vi "Controller Module.vi"(8 "error in":errorcluster) -> (0 "error out":errorcluster)   [LabVIEW 2025, in "Contoller.lvlib"]
doc: "This is the top level module for the ATM controller. \n\nIt is closed using a user event. It communicates with the other modules using aqueue based API which has comms modules that can be swapped if required."
uses:
  Contoller.lvlib
  Private Controls/Module Data Cluster.ctl
  Error Handler/Error Handler.lvlib
  Display/Display Console/Display Console.lvlib
  Public Control/ATM Transactions.ctl
  Private Controls/Control_Data.ctl
  Sensor/Sensor Console/Sensor Console.lvlib
  Simulated Console (UI)/Simulated Console.lvlib
  Config DataBase/Config Database.lvlib
  User Events/Controls/UE Abort Action.ctl
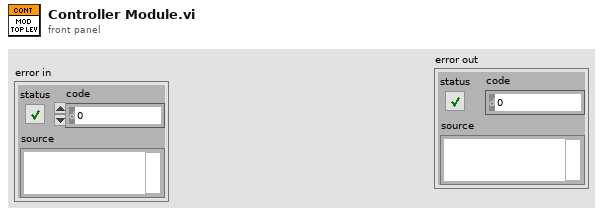
[diagram p1: front panel]
types:
  T1 = typedef "Contoller.lvlib/Control_Data.ctl" = cluster{"Transactions":T2, "Number Log Ins":dbl}
  T2 = typedef "Contoller.lvlib/ATM Transactions.ctl" = enum16{"Welcome", "Login", "Idle ", "Invalid Login", "Terminate Session", "Deposit", "Withdrawal", "Fast Cash", "Withdrawal Complete", "Withdrawal Failed", "Balance Inquiry"}
  T3 = typedef "Contoller.lvlib/Module Data Cluster.ctl" = cluster{"Data":variant, "Action":enum16{"Log In Init", "Fast Cash", "New transaction", "Withdrawal Init", "Recieve Keypad", "Deposit Finish", "Balance", "Withdrawal Approved", "Terminate", "Deposit Init", "Error", "Exit", "Init", "Log In Finish", "Cancel Transaction", "Withdrawal Failed", "Cash Removed"}}
  T4 = typedef "UE Abort Action.ctl" = enum16{"Destroy", "Get", "Create"}
  T5 = enum16{"Log In Init", "Fast Cash", "New transaction", "Withdrawal Init", "Recieve Keypad", "Deposit Finish", "Balance", "Withdrawal Approved", "Terminate", "Deposit Init", "Error", "Exit", "Init", "Log In Finish", "Cancel Transaction", "Withdrawal Failed", "Cash Removed"}
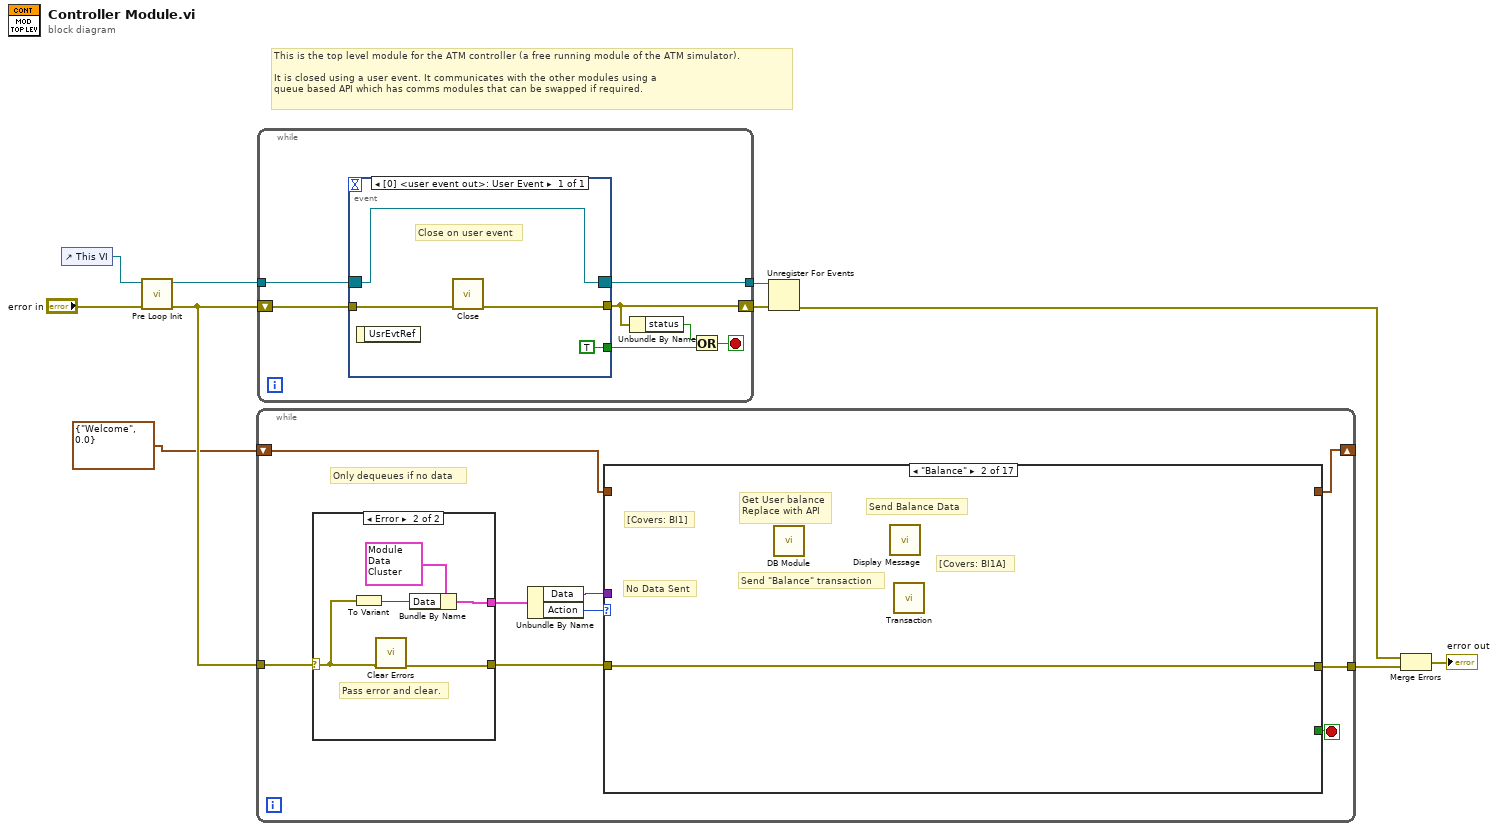
[diagram p0: block diagram]
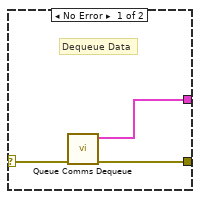
[diagram p2: hidden frame]
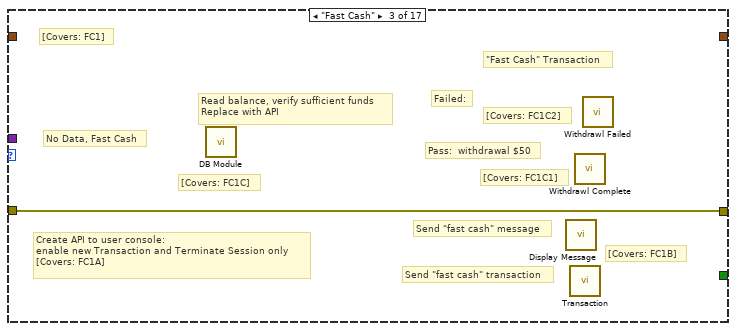
[diagram p4: hidden frame]
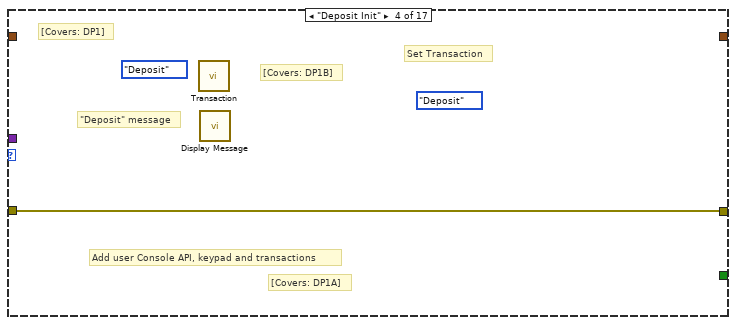
[diagram p5: hidden frame]
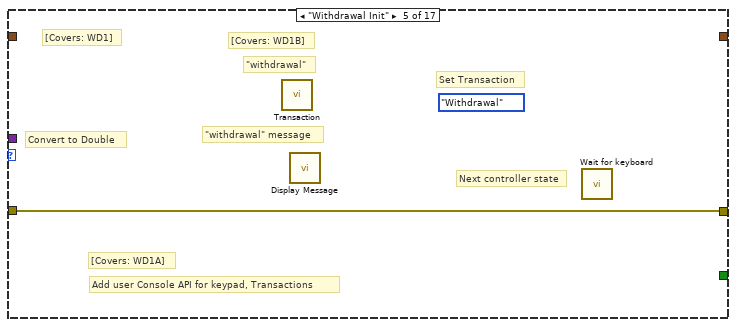
[diagram p6: hidden frame]
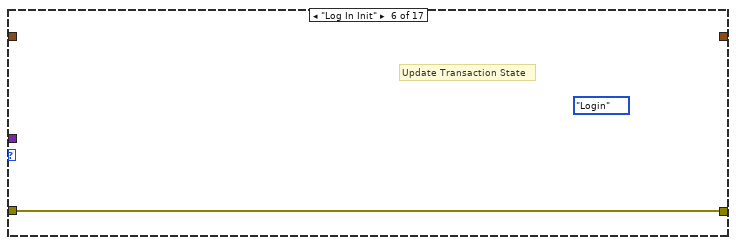
[diagram p7: hidden frame]
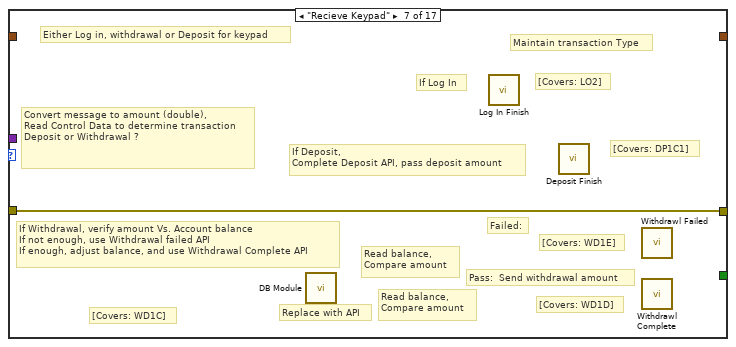
[diagram p8: hidden frame]
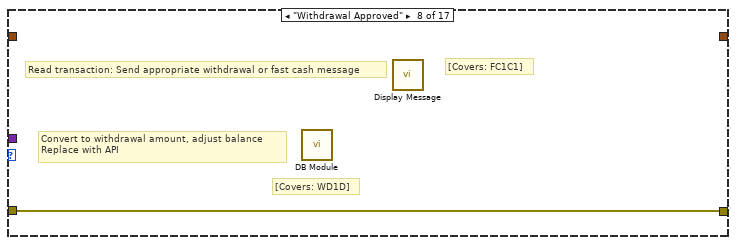
[diagram p9: hidden frame]
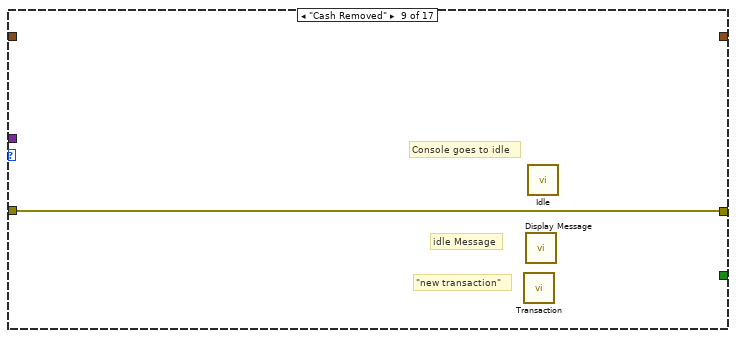
[diagram p10: hidden frame]
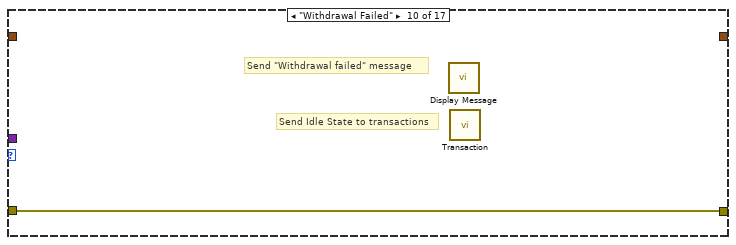
[diagram p11: hidden frame]
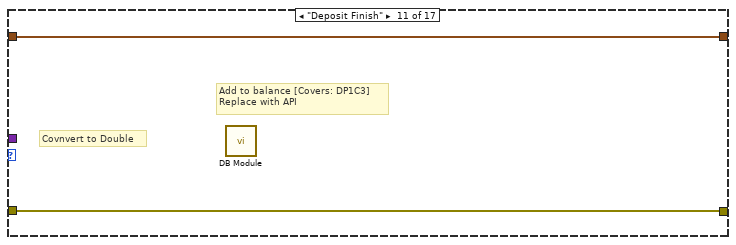
[diagram p12: hidden frame]
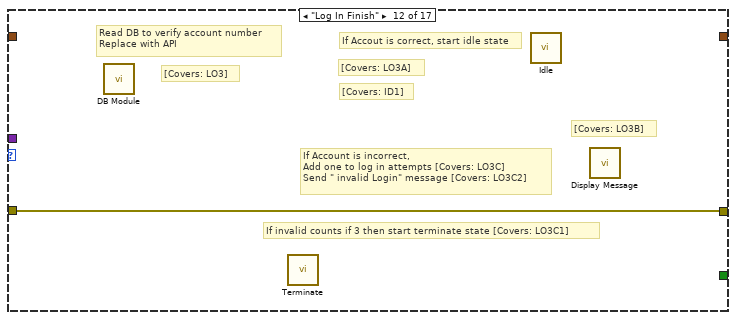
[diagram p13: hidden frame]
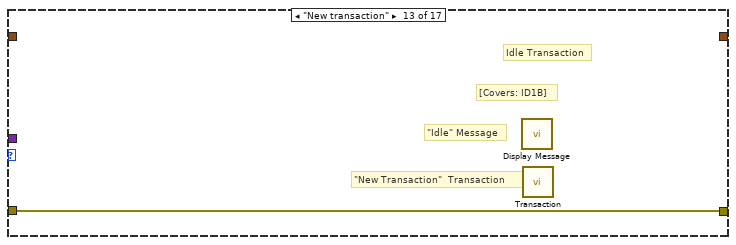
[diagram p14: hidden frame]
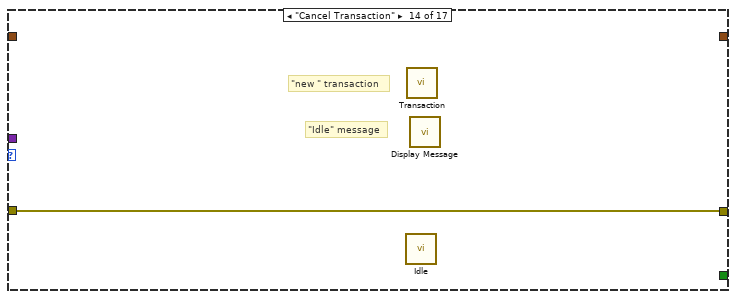
[diagram p15: hidden frame]
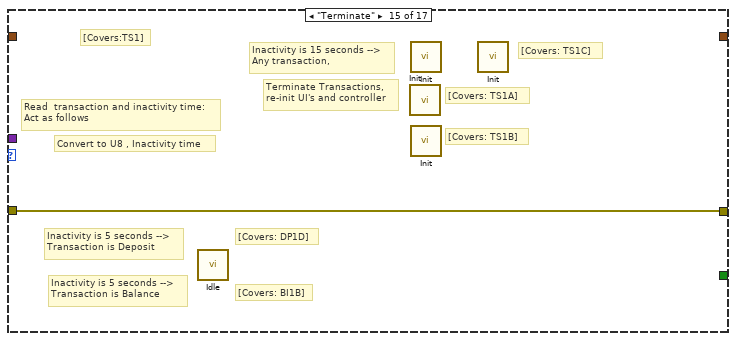
[diagram p16: hidden frame]
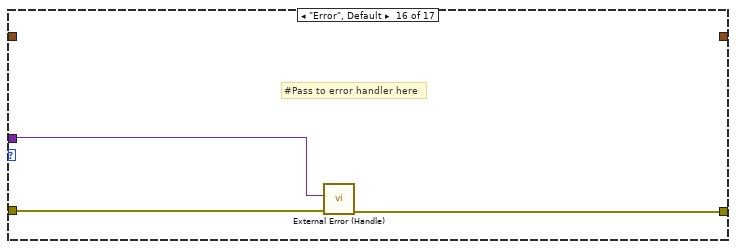
[diagram p17: hidden frame]
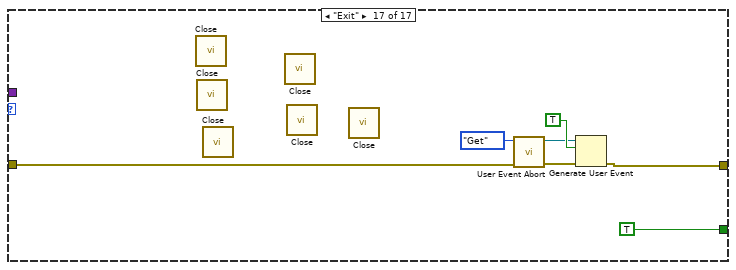
[diagram p18: hidden frame]
diagram:
  # "This is the top level module for the ATM controller (a free running module of the ATM simulator). \n\nIt is closed using a user event. It communicates with the other modules using a\nqueue based API which has comms modules that can be swapped if required."
  n1 = control-ref of="This VI"() -> (w10:refnum<vi>)
  n2 = call "Pre Loop Init.vi"("error in"="error in", "Ref In"=w10) -> ("error out"=w5:errorcluster, "Event Registration Refnum"=w8:refnum<event-registration>)  [unwired: 8 in]
  n3 = while {
    tunnel: w5 -> [w18]
    tunnel: [w13] -> w3
    shift-right: [w11] -> _
    shift-left: T1 {"Transactions"=enum."Welcome", "Number Log Ins"=0.0} ("Control_Data") -> [w12]
    stop <- w19 stop-if-true
    # "Only dequeues if no data"
    n4 = case shown="Error" w18 {
      selector: w18 -> [w21 w24]
      tunnel: [w22 w23] -> w16
      tunnel: [w20 w25] -> w17
      frame No Error {
        # "Dequeue Data"
        n5 = call "Queue Comms Dequeue.vi"("error in"=w21) -> ("error out"=w22:errorcluster, "Data Out"=w20:T3)  [unwired: 9 in]
      }
      frame Error {
        # "Pass error and clear."
        n6 = To Variant(anything=w24) -> (Variant=w26:variant)
        n7 = call <vilib>:"Clear Errors.vi"("error in (no error)"=w24) -> ("error out"=w23:errorcluster)  [unwired: 5 in, 1 out]
        n8 = Bundle By Name(cluster=T3 {"Data"=variant, "Action"=enum."Error"} ("Cluster"), "Data"=w26) -> (w25:T3)
      }
    }
    n9 = Unbundle By Name(w17) -> ("Data"=w14:variant, "Action"=w15:T5)
    n10 = case shown="\"Balance\"" w15 {
      tunnel: [_ _ _ _ _ _ _ _ _ _ _ _ _ _ _ _ TRUE] -> w19
      tunnel: w16 -> [w28 w29 w30 w31 w32 w33 w34 w35 w36 w37 w39 w40 w41 w42 w43 w45 w48]
      tunnel: w14 -> [_ _ _ _ _ _ _ _ _ _ _ _ _ _ _ w46 _]
      tunnel: [w28 w29 w30 w31 w32 w33 w34 w35 w36 w37 w39 w40 w41 w42 w43 w44 w47] -> w13
      tunnel: w12 -> [_ _ _ _ _ _ _ _ _ _ w38 _ _ _ _ _ _]
      tunnel: [_ _ _ _ _ _ _ _ _ _ w38 _ _ _ _ _ _] -> w11
      frame "Init" {
        # "Set Transaction to Init\nSet Log in attempts to 0"
      }
      frame "Balance" {
        # "[Covers: BI1A]"
        # "Send Balance Data"
        # "Send \"Balance\" transaction"
        # "Get User balance\nReplace with API"
        # "No Data Sent"
        # "[Covers: BI1]"
        n11 = call "DB Module.vi"() -> ()  [unwired: 11 in, 1 out]
        n12 = call "Display Message.vi"() -> ()  [unwired: 11 in, 1 out]
        n13 = call "Transaction.vi"() -> ()  [unwired: 11 in, 1 out]
      }
      frame "Fast Cash" {
        # "[Covers: FC1]"
        # "[Covers: FC1B]"
        # "Send \"fast cash\" transaction"
        # "Send \"fast cash\" message"
        # "\"Fast Cash\" Transaction"
        # "Create API to user console: \nenable new Transaction and Terminate Session only\n[Covers: FC1A]"
        # "[Covers: FC1C]"
        # "Failed:"
        # "[Covers: FC1C2]"
        # "[Covers: FC1C1]"
        # "Pass:  withdrawal $50"
        # "Read balance, verify sufficient funds\nReplace with API"
        # "No Data, Fast Cash"
        n14 = call "DB Module.vi"() -> ()  [unwired: 11 in, 1 out]
        n15 = call "Display Message.vi"() -> ()  [unwired: 11 in, 1 out]
        n16 = call "Transaction.vi"() -> ()  [unwired: 11 in, 1 out]
        n17 = call "Withdrawl Complete.vi"() -> ()  [unwired: 11 in, 1 out]
        n18 = call "Withdrawl Failed.vi"() -> ()  [unwired: 11 in, 1 out]
      }
      frame "Deposit Init" {
        (unwired) ATM_Transactions."Deposit" ("Transactions")
        (unwired) ATM_Transactions."Deposit" ("Transactions")
        # "[Covers: DP1]"
        # "Set Transaction"
        # "Add user Console API, keypad and transactions"
        # "[Covers: DP1A]"
        # "[Covers: DP1B]"
        # "\"Deposit\" message"
        n19 = call "Transaction.vi"() -> ()  [unwired: 11 in, 1 out]
        n20 = call "Display Message.vi"() -> ()  [unwired: 11 in, 1 out]
      }
      frame "Withdrawal Init" {
        (unwired) ATM_Transactions."Withdrawal" ("Transactions")
        # "[Covers: WD1]"
        # "Convert to Double"
        # "Next controller state"
        # "Add user Console API for keypad, Transactions"
        # "[Covers: WD1A]"
        # "Set Transaction"
        # "[Covers: WD1B]"
        # "\"withdrawal\""
        # "\"withdrawal\" message"
        n21 = call "Transaction.vi"() -> ()  [unwired: 11 in, 1 out]
        n22 = call "Display Message.vi"() -> ()  [unwired: 11 in, 1 out]
        n23 = call "Wait for keyboard.vi"() -> ()  [unwired: 11 in, 1 out]
      }
      frame "Log In Init" {
        (unwired) ATM_Transactions."Login" ("Transactions")
        # "Update Transaction State"
      }
      frame "Recieve Keypad" {
        # "Replace with API"
        # "Read balance,\nCompare amount"
        # "[Covers: WD1C]"
        # "[Covers: LO2]"
        # "If Log In"
        # "Failed:"
        # "[Covers: DP1C1]"
        # "Either Log in, withdrawal or Deposit for keypad"
        # "Maintain transaction Type"
        # "[Covers: WD1E]"
        # "[Covers: WD1D]"
        # "Read balance,\nCompare amount"
        # "Pass:  Send withdrawal amount"
        # "If Deposit, \nComplete Deposit API, pass deposit amount"
        # "If Withdrawal, verify amount Vs. Account balance\nIf not enough, use Withdrawal failed API\nIf enough, adjust balance, and use Withdrawal Complete API"
        # "Convert message to amount (double),\nRead Control Data to determine transaction\nDeposit or Withdrawal ?"
        n24 = call "DB Module.vi"() -> ()  [unwired: 11 in, 1 out]
        n25 = call "Log In Finish.vi"() -> ()  [unwired: 11 in, 1 out]
        n26 = call "Deposit Finish.vi"() -> ()  [unwired: 11 in, 1 out]
        n27 = call "Withdrawl Failed.vi"() -> ()  [unwired: 11 in, 1 out]
        n28 = call "Withdrawl Complete.vi"() -> ()  [unwired: 11 in, 1 out]
      }
      frame "Withdrawal Approved" {
        # "[Covers: FC1C1]"
        # "Read transaction: Send appropriate withdrawal or fast cash message"
        # "[Covers: WD1D]"
        # "Convert to withdrawal amount, adjust balance\nReplace with API"
        n29 = call "DB Module.vi"() -> ()  [unwired: 11 in, 1 out]
        n30 = call "Display Message.vi"() -> ()  [unwired: 11 in, 1 out]
      }
      frame "Cash Removed" {
        # "Console goes to idle"
        # "idle Message"
        # "\"new transaction\""
        n31 = call "Transaction.vi"() -> ()  [unwired: 11 in, 1 out]
        n32 = call "Display Message.vi"() -> ()  [unwired: 11 in, 1 out]
        n33 = call "Idle.vi"() -> ()  [unwired: 11 in, 1 out]
      }
      frame "Withdrawal Failed" {
        # "Send Idle State to transactions"
        # "Send \"Withdrawal failed\" message"
        n34 = call "Display Message.vi"() -> ()  [unwired: 11 in, 1 out]
        n35 = call "Transaction.vi"() -> ()  [unwired: 11 in, 1 out]
      }
      frame "Deposit Finish" {
        # "Add to balance [Covers: DP1C3]\nReplace with API"
        # "Covnvert to Double"
        n36 = call "DB Module.vi"() -> ()  [unwired: 11 in, 1 out]
      }
      frame "Log In Finish" {
        # "[Covers: ID1]"
        # "If invalid counts if 3 then start terminate state [Covers: LO3C1]"
        # "[Covers: LO3B]"
        # "If Account is incorrect, \nAdd one to log in attempts [Covers: LO3C] \nSend \" invalid Login\" message [Covers: LO3C2]"
        # "[Covers: LO3A]"
        # "If Accout is correct, start idle state"
        # "[Covers: LO3]"
        # "Read DB to verify account number\nReplace with API"
        n37 = call "DB Module.vi"() -> ()  [unwired: 11 in, 1 out]
        n38 = call "Terminate.vi"() -> ()  [unwired: 11 in, 1 out]
        n39 = call "Idle.vi"() -> ()  [unwired: 11 in, 1 out]
        n40 = call "Display Message.vi"() -> ()  [unwired: 11 in, 1 out]
      }
      frame "New transaction" {
        # "Idle Transaction"
        # "\"Idle\" Message"
        # "\"New Transaction\"  Transaction"
        # "[Covers: ID1B]"
        n41 = call "Display Message.vi"() -> ()  [unwired: 11 in, 1 out]
        n42 = call "Transaction.vi"() -> ()  [unwired: 11 in, 1 out]
      }
      frame "Cancel Transaction" {
        # "\"Idle\" message"
        # "\"new \" transaction"
        n43 = call "Idle.vi"() -> ()  [unwired: 11 in, 1 out]
        n44 = call "Transaction.vi"() -> ()  [unwired: 11 in, 1 out]
        n45 = call "Display Message.vi"() -> ()  [unwired: 11 in, 1 out]
      }
      frame "Terminate" {
        # "[Covers:TS1]"
        # "Inactivity is 5 seconds -->\nTransaction is Balance"
        # "[Covers: BI1B]"
        # "[Covers: DP1D]"
        # "Inactivity is 5 seconds -->\nTransaction is Deposit"
        # "Inactivity is 15 seconds -->\nAny transaction,"
        # "Convert to U8 , Inactivity time"
        # "Read  transaction and inactivity time:\nAct as follows"
        # "[Covers: TS1C]"
        # "[Covers: TS1B]"
        # "[Covers: TS1A]"
        # "Terminate Transactions, \nre-init UI's and controller"
        n46 = call "Idle.vi"() -> ()  [unwired: 11 in, 1 out]
        n47 = call "Init.vi"() -> ()  [unwired: 11 in, 1 out]
        n48 = call "Init.vi"() -> ()  [unwired: 11 in, 1 out]
        n49 = call "Init.vi"() -> ()  [unwired: 11 in, 1 out]
        n50 = call "Init.vi"() -> ()  [unwired: 11 in, 1 out]
      }
      frame "Error", Default {
        # "#Pass to error handler here"
        n51 = call "External Error (Handle).vi"("error in"=w45, "Data"=w46) -> ("error out"=w44:errorcluster)  [unwired: 9 in]
      }
      frame "Exit" {
        n52 = call "Close.vi"() -> ()  [unwired: 11 in, 1 out]
        n53 = call "Close.vi"() -> ()  [unwired: 11 in, 1 out]
        n54 = call "Close.vi"() -> ()  [unwired: 11 in, 1 out]
        n55 = call "Close.vi"() -> ()  [unwired: 11 in, 1 out]
        n56 = call "Close.vi"() -> ()  [unwired: 11 in, 1 out]
        n57 = call "Close.vi"() -> ()  [unwired: 11 in, 1 out]
        n58 = call "User Event Abort.vi"("error in"=w48, "Action"=UE_Abort_Action."Get") -> ("error out"=w50:errorcluster, "user event out"=w51:refnum<user-event>)  [unwired: 8 in]
        n59 = Generate User Event(user event=w51, event data cluster=TRUE ("event data"), error in=w50) -> (error out=w47:errorcluster)  [unwired: 1 in, 1 out]
      }
    }
  }
  n60 = while {
    shift-right: [w57] -> w7
    shift-left: w5 -> [w60]
    tunnel: w8 -> [w55]
    tunnel: [w54] -> w6
    stop <- w58 stop-if-true
    n61 = event shown="[0] <user event out>: User Event" {
      selector: w55 -> [w64]
      dyn-events: [w64] -> w54
      timeout: _ -> [_]
      tunnel: w60 -> [w63]
      tunnel: [w62] -> w57
      tunnel: [TRUE ("stop")] -> w59
      event User Event {
        # "Close on user event"
        n62 = event-data() -> ()  [unwired: 1 in, 1 out]
        n63 = call "Close.vi"("error in"=w63) -> ("error out"=w62:errorcluster)  [unwired: 10 in]
      }
    }
    n64 = Unbundle By Name(w57) -> ("status"=w56:bool)
    n65 = Or(x=w56, y=w59) -> (x .or. y?=w58:bool)
  }
  n66 = Unregister For Events(event registration refnum=w6, error in=w7) -> (error out=w2:errorcluster)
  n67 = Merge Errors(w2, w3) -> (→"error out":errorcluster)
